vi "New.vi"(8 "error in (no error)":errorcluster, 11 "ByRefClass in":refnum<class "ClassByRef.lvclass">) -> (0 "error out":errorcluster, 3 "ByRefClass out":refnum<class "ClassByRef.lvclass">)   [LabVIEW 2021, in "ClassUtilities.lvlib" / "ClassByRef.lvclass"]
uses:
  ClassByRef.lvclass
  ClassByRef.lvclass/ClassByRef.ctl
  SetRef.vi
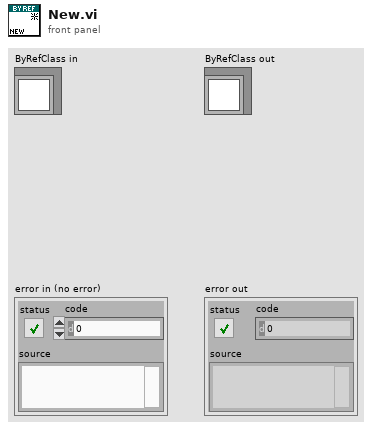
[diagram p1: front panel]
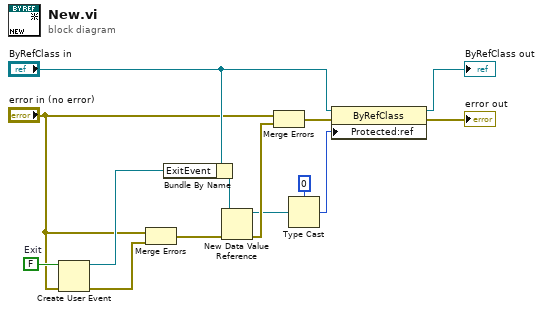
[diagram p0: block diagram]
diagram:
  w5 = FALSE  # Exit
  n1 = Create User Event(user event datatype=w5, error in="error in (no error)") -> (user event=w4:refnum<user-event>, error out=w2:errorcluster)
  n2 = Merge Errors("error in (no error)", w2) -> (w3:errorcluster)
  n3 = Bundle By Name(cluster="ByRefClass in", "ExitEvent"=w4) -> (w6:refnum<class "ClassByRef.lvclass">)
  n4 = New Data Value Reference(data value=w6, error in=w3) -> (data value reference=w13:refnum<data-value>, error out=w14:errorcluster)
  n5 = Merge Errors("error in (no error)", w14) -> (w10:errorcluster)
  n6 = Type Cast(type=u64 0, x=w13) -> (*(type *) &x=w11:u64)
  n7 = property class="ByRefClass"(reference="ByRefClass in", error in=w10, "Protected:ref"=w11) -> (reference out=→"ByRefClass out":refnum<class "ClassByRef.lvclass">, error out=→"error out":errorcluster)
